vi "Thermal Chamber Controller with Multiple DUTs.vi"() -> ()   [LabVIEW 2015]
doc: "Implements a Thermal Chamber Controller with multiple DUTs, using a <b>singleton</b> Delacor QMH Module for the controller, and multiple instances of a <b>cloneable</b> Delacor QMH module for the DUT. The chamber is configured to reach a temperature set point. Once the temperature is reached, multiple Units Under Test (UUTs) each perform a Self Test and return the result. The Unit Under Test code is configured for an 80% pass rate for demonstration purposes.\n\nThis example illustrates that there is no need to have an event structure in the calling code and provides an example of two DQMH modules being used in a traditional \"Configure > Read/Write > Close\" application. The example also illustrates how to manage multiple instances of a cloneable DQMH module.\n____\nDelacor QMH Thermal Chamber Examples 4.0.0.21\nCopyright (c) 2018, Delacor"
uses:
  Libraries/Thermal Chamber Controller_DQMH/Heater State--enum.ctl
  Libraries/Thermal Chamber Controller_DQMH/Thermal Chamber Controller_DQMH.lvlib
  Libraries/Device Under Test_Cloneable_DQMH/Device Under Test_Cloneable_DQMH.lvlib
panel:
  in  "Number of DUTs":i32=5
  out "Self Test Results":bool[](array[boolean])
  # "Overview: Demonstrates how to implement a Thermal Chamber Controller with multiple DUTs, using a singleton Delacor QMH Module for the controller, and multiple instances of a cloneable Delacor QMH module for the DUTs.\nRequirements: Delacor QMH\nInstructions:\n1. Make sure you are already familiar with the concepts described in the Thermal Chamber Controller.vi and Thermal Chamber Controller with DUT.vi examples in the DQMH Fundamentals project.\n2. Run this VI to launch the singleton Thermal Chamber Controller DQMH module and multiple instances of the Device Under Test DQMH module.\n3. Observe the temperature in the Thermal Chamber rise as it approaches the set point.\n4. Once the temperature has been reached, observe that the DUT test simulations start. You can move the front panels of the DUT instances to different positions as they appear if you wish to see more than one at a time.\n5. Once the DUT tests are complete, the example will stop. See the block diagram of this VI for more information."
  # "(The DUT simulator has a self test pass rate of 80%)."
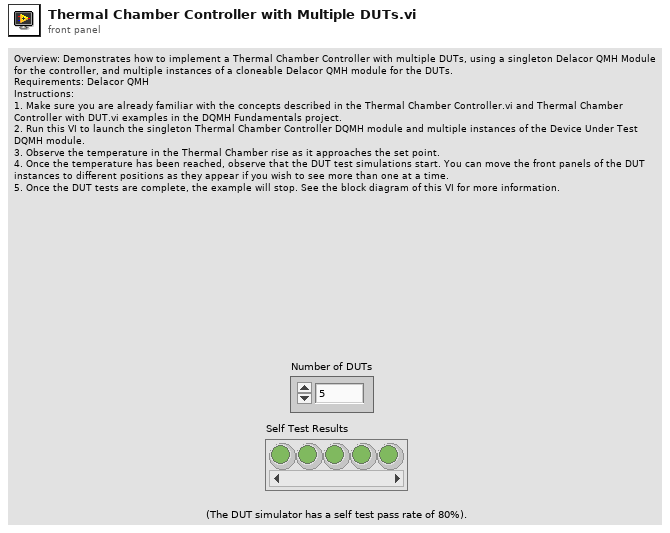
[diagram p1: front panel]
types:
  T1 = typedef "Thermal Chamber Controller_DQMH.lvlib/Heater State--enum.ctl" = enum16{"Heater Enabled", "Heater Disabled"}
  T2 = typedef "Thermal Chamber Controller_DQMH.lvlib/Request and Wait for Status (Reply Payload)--cluster.ctl" = cluster{"Actual Temperature":dbl, "Temperature Set Point":dbl, "Temperature Ramp Rate":dbl, "Heater State":T1, "error":errorcluster}
  T3 = typedef "Device Under Test_Cloneable_DQMH.lvlib/Perform Self Test (Reply Payload)--cluster.ctl" = cluster{"Result":bool, "error":errorcluster}
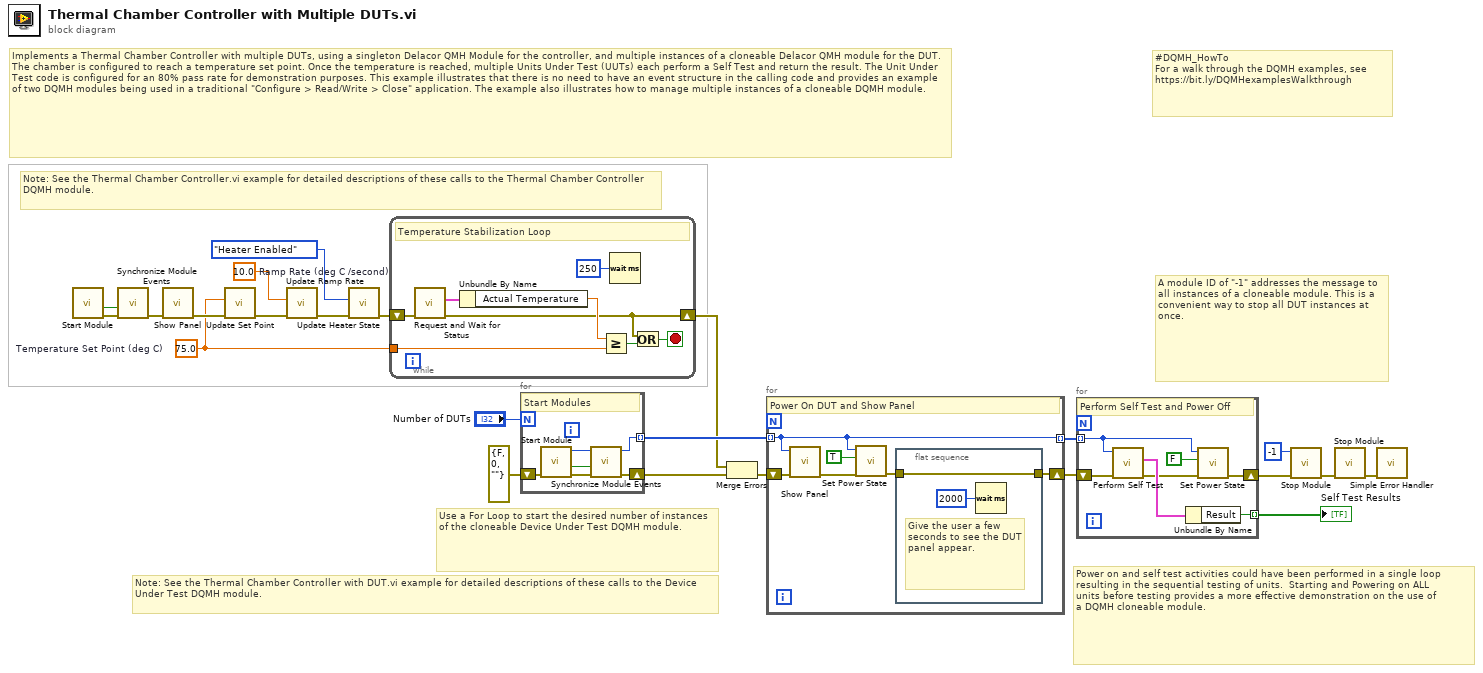
[diagram p0: block diagram]
diagram:
  w8 = 10.0  # Ramp Rate (deg C /second)
  w7 = 75.0  # Temperature Set Point (deg C)
  # "#DQMH_HowTo \nFor a walk through the DQMH examples, see https://bit.ly/DQMHexamplesWalkthrough"
  # "Use a For Loop to start the desired number of instances of the cloneable Device Under Test DQMH module."
  # "A module ID of \"-1\" addresses the message to all instances of a cloneable module. This is a convenient way to stop all DUT instances at once."
  # "Note: See the Thermal Chamber Controller with DUT.vi example for detailed descriptions of these calls to the Device Under Test DQMH module."
  # "Note: See the Thermal Chamber Controller.vi example for detailed descriptions of these calls to the Thermal Chamber Controller DQMH module."
  # "Implements a Thermal Chamber Controller with multiple DUTs, using a singleton Delacor QMH Module for the controller, and multiple instances of a cloneable Delacor QMH module for the DUT. The chamber is configured to reach a temperature set point. Once the temperature is reached, multiple Units Under Test (UUTs) each perform a Self Test and return the result. The Unit Under Test code is configured for an 80% pass rate for demonstration purposes. This example illustrates that there is no need to have an event structure in the calling code and provides an example of two DQMH modules being used in a traditional \"Configure > Read/Write > Close\" application. The example also illustrates how to manage multiple instances of a cloneable DQMH module."
  # "Power on and self test activities could have been performed in a single loop\nresulting in the sequential testing of units.  Starting and Powering on ALL \nunits before testing provides a more effective demonstration on the use of \na DQMH cloneable module."
  n1 = call "Start Module.vi"() -> ("error out"=w12:errorcluster, "Wait for Event Sync?"=w9:bool)  [unwired: 8 in, 2 out]
  n2 = call "Synchronize Module Events.vi"("error in (no error)"=w12, "Wait for Event Sync?"=w9) -> ("error out"=w11:errorcluster)  [unwired: 9 in]
  n3 = call "Show Panel.vi"("error in (no error)"=w11) -> ("error out"=w10:errorcluster)  [unwired: 10 in]
  n4 = call "Update Set Point.vi"("error in (no error)"=w10, "Temperature Set Point"=w7) -> ("error out"=w14:errorcluster)  [unwired: 9 in]
  n5 = call "Update Ramp Rate.vi"("error in (no error)"=w14, "Temperature Ramp Rate"=w8) -> ("error out"=w13:errorcluster)  [unwired: 9 in]
  n6 = call "Update Heater State.vi"("error in (no error)"=w13, "Heater State"=Heater_State--enum."Heater Enabled") -> ("error out"=w15:errorcluster)  [unwired: 9 in]
  n7 = while {
    shift-right: [w24] -> w6
    shift-left: w15 -> [w29]
    tunnel: w7 -> [w31]
    stop <- w26 stop-if-true
    # "Temperature Stabilization Loop"
    n8 = call "Request and Wait for Status.vi"("error in (no error)"=w29) -> ("error out"=w24:errorcluster, "Reply Payload"=w28:T2)  [unwired: 8 in, 1 out]
    n9 = Unbundle By Name(w28) -> ("Actual Temperature"=w30:dbl)
    n10 = Greater Or Equal?(x=w30, y=w31) -> (x >= y?=w25:bool)
    n11 = Wait (ms)(milliseconds to wait=u32 250) -> ()  [unwired: 1 out]
    n12 = Or(x=w24, y=w25) -> (x .or. y?=w26:bool)
  }
  n13 = for {
    N: "Number of DUTs" -> [_]
    tunnel: [w34] -> w20 mode=indexing
    shift-right: [w36] -> w22
    shift-left: errorcluster {"status"=FALSE, "code"=0, "source"=""} ("error constant") -> [w32]
    # "Start Modules"
    n14 = call "Start Module.vi"("error in (no error)"=w32) -> ("error out"=w33:errorcluster, "Wait for Event Sync?"=w37:bool, "Module ID"=w35:i32)  [unwired: 7 in, 1 out]
    n15 = call "Synchronize Module Events.vi"("error in (no error)"=w33, "Wait for Event Sync?"=w37, "Module ID"=w35) -> ("error out"=w36:errorcluster, "Module ID (dup)"=w34:i32)  [unwired: 7 in]
  }
  n16 = Merge Errors(w6, w22) -> (w23:errorcluster)
  n17 = for {
    tunnel: w20 -> [w38] mode=indexing
    shift-right: [w39] -> w18
    shift-left: w23 -> [w43]
    tunnel: [w38] -> w19 mode=indexing
    # "Power On DUT and Show Panel"
    n18 = call "Show Panel.vi"("error in (no error)"=w43, "Module ID"=w38) -> ("error out"=w41:errorcluster)  [unwired: 9 in]
    n19 = call "Set Power State.vi"("error in (no error)"=w41, "Power State"=TRUE, "Module ID"=w38) -> ("error out"=w40:errorcluster)  [unwired: 8 in]
    n20 = flat-sequence {
      tunnel: w40 -> [w45]
      tunnel: [w45] -> w39
      frame #0 {
        # "Give the user a few seconds to see the DUT panel appear."
        n21 = Wait (ms)(milliseconds to wait=u32 2000) -> ()  [unwired: 1 out]
      }
    }
  }
  n22 = for {
    shift-right: [w48] -> w16
    shift-left: w18 -> [w52]
    tunnel: w19 -> [w47] mode=indexing
    tunnel: [w50] -> w17 mode=indexing
    # "Perform Self Test and Power Off"
    n23 = call "Perform Self Test.vi"("error in (no error)"=w52, "Module ID"=w47) -> ("error out"=w46:errorcluster, "Reply Payload"=w51:T3)  [unwired: 7 in, 1 out]
    n24 = Unbundle By Name(w51) -> ("Result"=w50:bool)
    n25 = call "Set Power State.vi"("error in (no error)"=w46, "Power State"=FALSE, "Module ID"=w47) -> ("error out"=w48:errorcluster)  [unwired: 8 in]
  }
  "Self Test Results" <- w17
  n26 = call "Stop Module.vi"("error in (no error)"=w16, "Module ID"=-1) -> ("error out"=w3:errorcluster)  [unwired: 9 in]
  n27 = call "Stop Module.vi"("error in (no error)"=w3) -> ("error out"=w2:errorcluster)  [unwired: 10 in]
  n28 = call <vilib>:"Simple Error Handler.vi"("error in (no error)"=w2) -> ()  [unwired: 4 in, 5 out]
